vi "InsertMeasurementJsonConverter.vi"() -> ()   [LabVIEW 2012, in "LotData.lvclass"]
uses:
  LotData.lvclass
  Controls/JsonTypes/InsertMeasurement.ctl
  Controls/MeasurementType.ctl
panel:
  in  "InsertMeasurement":T1
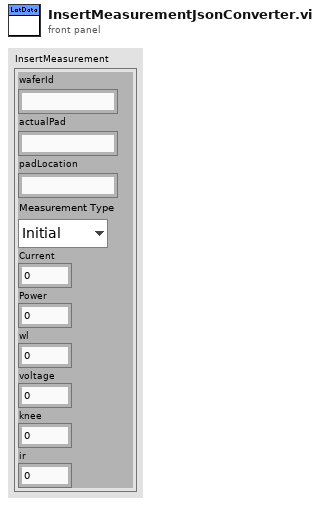
[diagram p1: front panel]
types:
  T1 = typedef "InsertMeasurement.ctl" = cluster{"waferId":string, "actualPad":string, "padLocation":string, "Measurement Type":T2, "Current":dbl, "Power":dbl, "wl":dbl, "voltage":dbl, "knee":dbl, "ir":dbl}
  T2 = typedef "MeasurementType.ctl" = enum16{"Initial", "Final"}
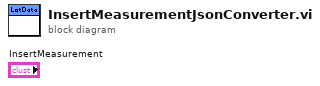
[diagram p0: block diagram]
diagram:
